vi "Load Contestant Panel.vi"(8 "error in (no error)":errorcluster, 9 "VI Ref":refnum<vi>, 10 "Contestant":i32, 11 "Controller in":refnum<class "Controller.lvclass">) -> (0 "error out":errorcluster, 3 "Controller out":refnum<class "Controller.lvclass">)   [LabVIEW 2021, in "Controller.lvlib" / "Controller.lvclass"]
uses:
  Controller.lvclass
  Controller.lvclass/Controller.ctl
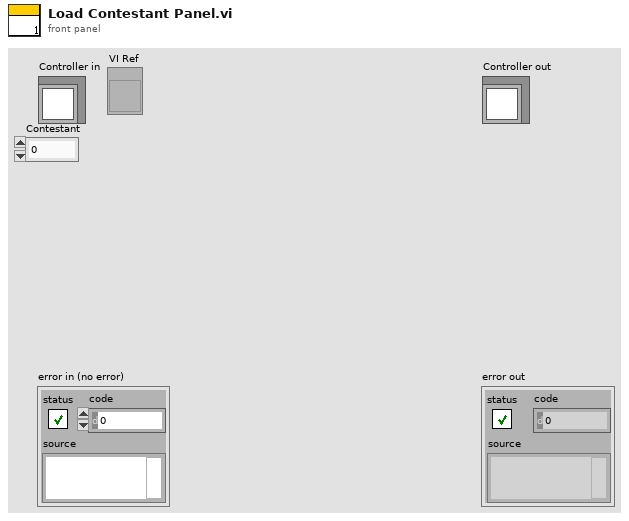
[diagram p1: front panel]
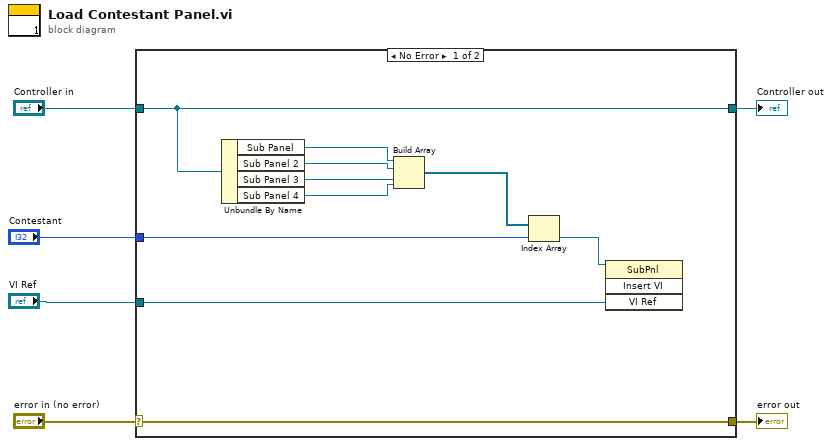
[diagram p0: block diagram]
diagram:
  n1 = case shown="No Error" "error in (no error)" {
    selector: "error in (no error)" -> [w16 w18]
    tunnel: [w16 w18] -> w5
    tunnel: [w15 w17] -> w3
    tunnel: "Controller in" -> [w15 w17]
    tunnel: "Contestant" -> [w9 _]
    tunnel: "VI Ref" -> [w7 _]
    frame No Error {
      n2 = Unbundle By Name(w15) -> ("Sub Panel"=w11:refnum<vi>, "Sub Panel 2"=w12:refnum<vi>, "Sub Panel 3"=w13:refnum<vi>, "Sub Panel 4"=w14:refnum<vi>)
      n3 = Build Array(w11, w12, w13, w14) -> (w10:refnum<vi>[])
      n4 = Index Array(array=w10, index=w9) -> (element=w8:refnum<vi>)
      n5 = invoke on="Invoke Node" class="SubPnl" method="Insert VI"(reference=w8, "VI Ref"=w7) -> ()  [unwired: 2 in, 4 out]
    }
    frame Error {
    }
  }
  "error out" <- w5
  "Controller out" <- w3
